vi "PAN_MacroReadCmds.vi"(10 "CommandStr":string, 11 "macrodir":path) -> (1 "macro":path, 2 "commands":string[](array[string]), 3 "macro":bool)   [LabVIEW 2016]
panel:
  out "output path":path
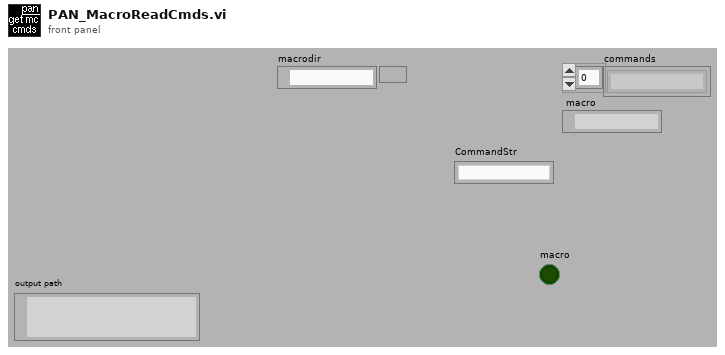
[diagram p1: front panel]
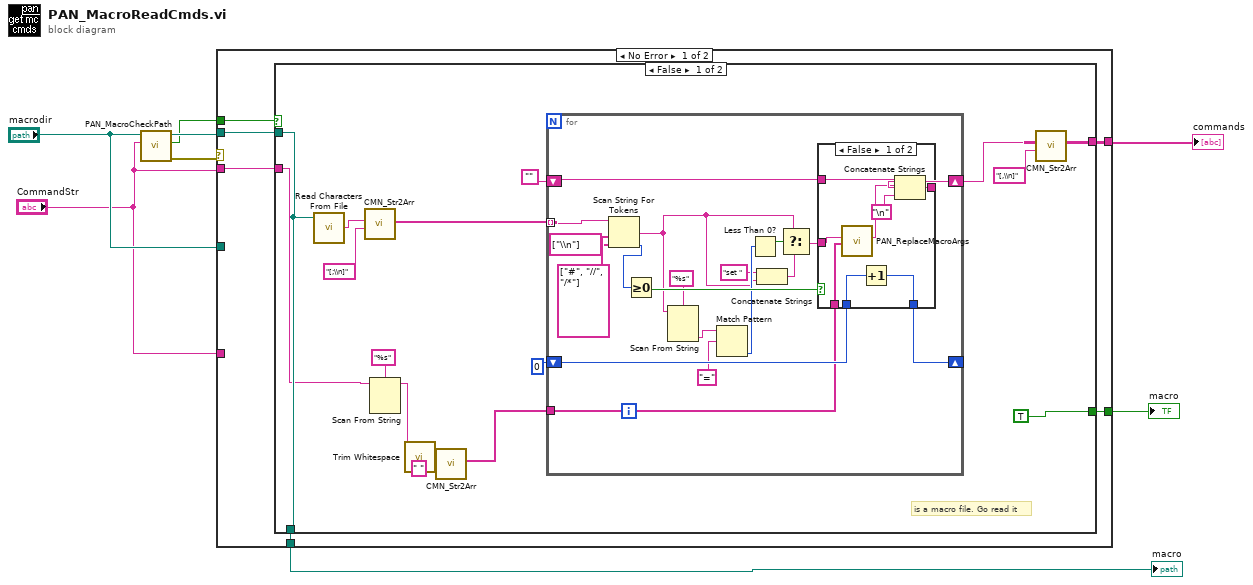
[diagram p0: block diagram]
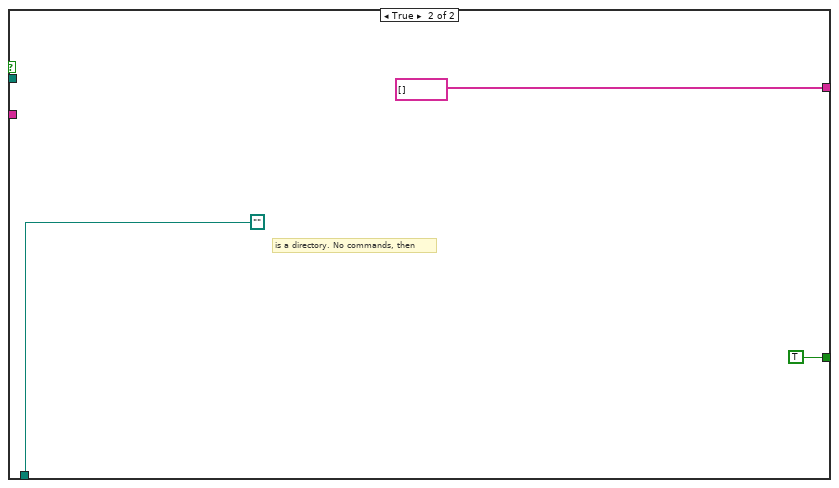
[diagram p3: hidden frame]
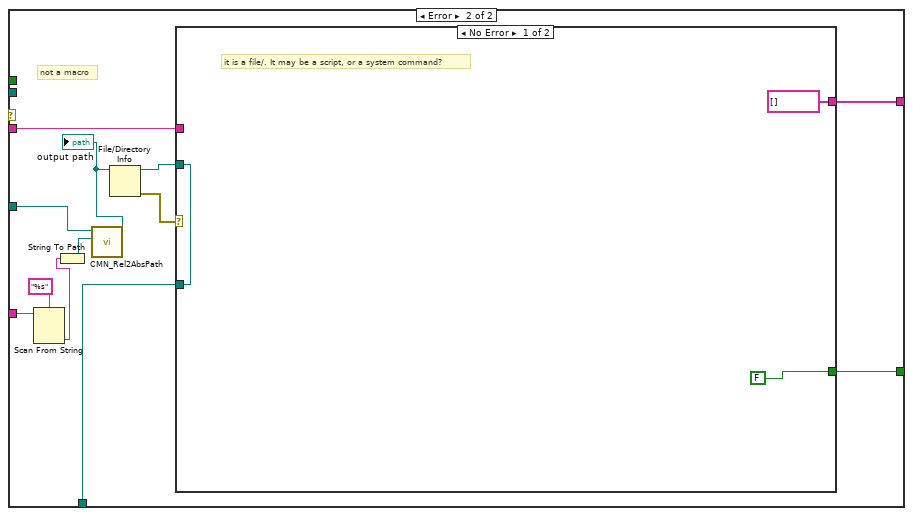
[diagram p4: hidden frame]
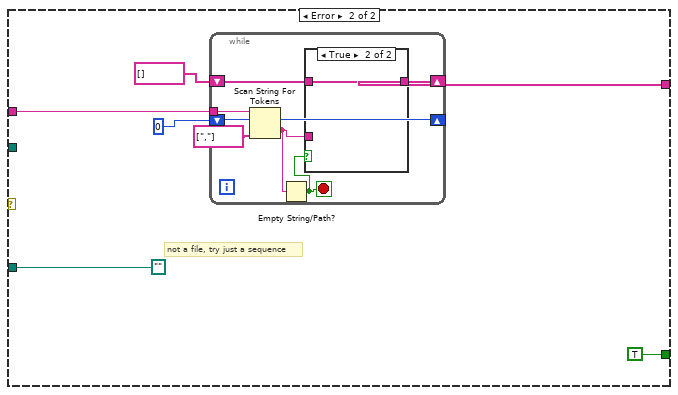
[diagram p5: hidden frame]
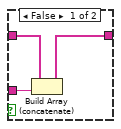
[diagram p6: hidden frame]
diagram:
  n1 = call "PAN_MacroCheckPath.vi"("CommandStr"="CommandStr", "macrodir"="macrodir") -> ("error out"=w6:errorcluster, "dir?"=w4:bool, "output path"=w5:path)  [unwired: 7 out]
  n2 = case shown="No Error" w6 {
    tunnel: "CommandStr" -> [w10 w74]
    tunnel: [w13 w73] -> w8
    tunnel: w4 -> [w14 _]
    tunnel: w5 -> [w12 _]
    tunnel: [w11 w72] -> w7
    tunnel: [w9 w63] -> w3
    tunnel: "macrodir" -> [_ w70]
    tunnel: "CommandStr" -> [_ w68]
    frame No Error {
      n3 = case shown="False" w14 {
        tunnel: [w30 string[] []] -> w13
        tunnel: w12 -> [w29 _]
        tunnel: [w29 path ""] -> w11
        tunnel: w10 -> [w26 _]
        tunnel: [TRUE ("macro") TRUE ("macro")] -> w9
        frame False {
          # "is a macro file. Go read it"
          n4 = call <vilib>:"Read Characters From File.vi"("file path (dialog if empty)"=w29) -> ("character string"=w28:string)  [unwired: 1 in, 7 out]
          n5 = call "CMN_Str2Arr.vi"("separator"="[;\\n]", "string in"=w28) -> ("Array out"=w25:string[])  [unwired: 2 in, 7 out]
          n6 = Scan From String(format string="%s", input string=w26) -> (remaining string=w17:string)  [unwired: 2 in, 4 out]
          n7 = call <vilib>:"Trim Whitespace.vi"("string"=w17) -> ("trimmed string"=w16:string)  [unwired: 1 in]
          n8 = call "CMN_Str2Arr.vi"("separator"=" ", "string in"=w16) -> ("Array out"=w19:string[])  [unwired: 2 in, 7 out]
          n9 = for {
            tunnel: w25 -> [w49] mode=indexing
            shift-right: [w40] -> w15
            shift-left: "" -> [w47]
            shift-right: [w43] -> _
            shift-left: 0 -> [w42]
            tunnel: w19 -> [w41]
            n10 = Scan String For Tokens(6:string[] ["\\n"] ("delimiters (\\s,\\t,\\r,\\n)"), 7:string[] ["#", "//", "/*"] ("operators (none)"), 9:w49) -> (0:w45:i32, 1:w33:string)  [unwired: 1 in, 4 out]
            n11 = Greater Or Equal To 0?(x=w45) -> (x >= 0?=w44:bool)
            n12 = Scan From String(format string="%s", input string=w33) -> (output 1=w38:string)  [unwired: 2 in, 4 out]
            n13 = Match Pattern(string=w38, regular expression="=") -> (offset past match=w36:i32)  [unwired: 4 out]
            n14 = Less Than 0?(x=w36) -> (x < 0?=w32:bool)
            n15 = Concatenate Strings("set " ("string"), w33) -> (w31:string)
            n16 = Select(t=w33, s=w32, f=w31) -> (s? t:f=w35:string)
            n17 = case shown="False" w44 {
              tunnel: [w57 w59] -> w40
              tunnel: w35 -> [w52 _]
              tunnel: w47 -> [w55 w59]
              tunnel: w42 -> [w54 w58]
              tunnel: [w53 w58] -> w43
              tunnel: w41 -> [w50 _]
              frame False {
                n18 = call "PAN_ReplaceMacroArgs.vi"("args"=w50, "command in"=w52) -> ("comand out"=w51:string)  [unwired: 9 out]
                n19 = Increment(x=w54) -> (x+1=w53:i32)
                n20 = Concatenate Strings(w55, w51, "\n") -> (w57:string)
              }
              frame True {
              }
            }
          }
          n21 = call "CMN_Str2Arr.vi"("separator"="[,\\n]", "string in"=w15) -> ("Array out"=w30:string[])  [unwired: 2 in, 7 out]
        }
        frame True {
          # "is a directory. No commands, then"
        }
      }
    }
    frame Error {
      # "not a macro"
      n22 = Scan From String(format string="%s", input string=w68) -> (output 1=w67:string)  [unwired: 2 in, 4 out]
      n23 = String To Path(string=w67) -> (path=w66:path)
      n24 = call "CMN_Rel2AbsPath.vi"("test path"=w66, "absolute path"=w70) -> ("output path"=w71:path)  [unwired: 1 in, 8 out]
      "output path" <- w71
      n25 = File/Directory Info(path=w71) -> (path out=w64:path, error out=w65:errorcluster)  [unwired: 1 in, 5 out]
      n26 = case shown="No Error" w65 {
        tunnel: w74 -> [_ w83]
        tunnel: [string[] [] w80] -> w73
        tunnel: [w77 path ""] -> w72
        tunnel: w64 -> [w77 _]
        tunnel: [FALSE ("macro") TRUE ("macro")] -> w63
        frame No Error {
          # "it is a file/. It may be a script, or a system command?"
        }
        frame Error {
          # "not a file, try just a sequence"
          n27 = while {
            shift-left: 0 -> [w88]
            shift-right: [w87] -> _
            tunnel: w83 -> [w89]
            shift-left: string[] [] -> [w85]
            shift-right: [w91] -> w80
            stop <- w84 stop-if-true
            n28 = Scan String For Tokens(6:string[] [","] ("delimiters (\\s,\\t,\\r,\\n)"), 8:w88, 9:w89) -> (1:w86:string, 2:w87:i32)  [unwired: 5 out]
            n29 = Empty String/Path?(string/path=w86) -> (empty?=w84:bool)
            n30 = case shown="True" w84 {
              tunnel: [w94 w95] -> w91
              tunnel: w86 -> [w93 _]
              tunnel: w85 -> [w92 w95]
              frame False {
                n31 = Build Array (concatenate)(w92, w93) -> (w94:string[])
              }
              frame True {
              }
            }
          }
        }
      }
    }
  }
  "commands" <- w8
  "macro" <- w7
  "macro" <- w3
